vi "Tosca-Compute Histogram.vi"(0 "Results in":T1[](array[typedef]), 5 "family":string, 7 "Result String":string, 9 "Result":T2) -> (4 "Results out":T1[](array[typedef]))   [LabVIEW 2020]
uses:
  Classes/Parameters/Histogram Data.ctl
  Typedefs/Tosca-Trial Result Enum.ctl
  Classes/Parameters/Parameters.lvclass
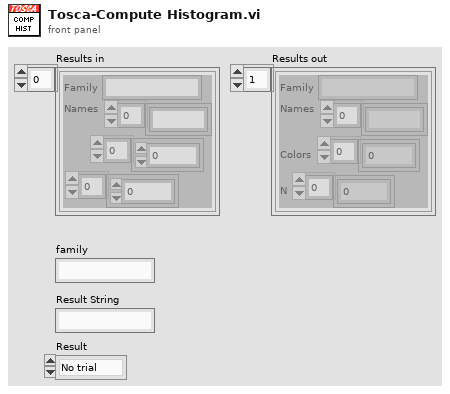
[diagram p1: front panel]
types:
  T1 = typedef "Parameters.lvclass/Histogram Data.ctl" = cluster{"Family":string, "Names":string[], "Colors":u32[], "N":i32[]}
  T2 = typedef "Tosca-Trial Result Enum.ctl" = enum16{"No trial", "Go", "No go", "Error", "Abort"}
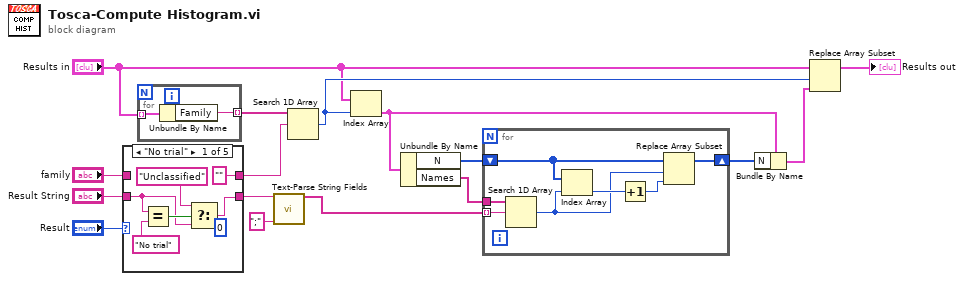
[diagram p0: block diagram]
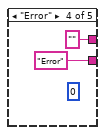
[diagram p4: hidden frame]
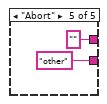
[diagram p5: hidden frame]
diagram:
  n1 = case shown="\"No trial\"" "Result" {
    tunnel: [w20 w23 w25 "Error" ("family") "other" ("family")] -> w6
    tunnel: "family" -> [_ w24 w26 _ _]
    tunnel: ["" ("family") w24 w26 "" ("family") "" ("family")] -> w11
    tunnel: "Result String" -> [w18 w23 w25 _ _]
    frame "No trial" {
      (unwired) i16 0
      n2 = Equal?(x=w18, y="No trial" ("family")) -> (x = y?=w19:bool)
      n3 = Select(t="Unclassified" ("family"), s=w19, f=w18) -> (s? t:f=w20:string)
    }
    frame "Go", Default {
    }
    frame "No go" {
    }
    frame "Error" {
      (unwired) i16 0
    }
    frame "Abort" {
    }
  }
  n4 = for {
    tunnel: "Results in" -> [w32] mode=indexing
    tunnel: [w31] -> w1 mode=indexing
    n5 = Unbundle By Name(w32) -> ("Family"=w31:string)
  }
  n6 = call "Text-Parse String Fields.vi"("String"=w6, "Separator"=";") -> ("Fields"=w4:string[])  [unwired: 8 in, 5 out]
  n7 = Search 1D Array(1D array=w1, element=w11) -> (index of element=w3:i32)  [unwired: 1 in]
  n8 = Index Array(array="Results in", index=w3) -> (element=w9:T1)
  n9 = Unbundle By Name(w9) -> ("N"=w7:i32[], "Names"=w8:string[])
  n10 = for {
    tunnel: w8 -> [w36]
    shift-right: [w39] -> w13
    shift-left: w7 -> [w35]
    tunnel: w4 -> [w33] mode=indexing
    n11 = Search 1D Array(1D array=w36, element=w33) -> (index of element=w34:i32)  [unwired: 1 in]
    n12 = Index Array(array=w35, index=w34) -> (element=w38:i32)
    n13 = Increment(x=w38) -> (x+1=w37:i32)
    n14 = Replace Array Subset(array=w35, new element=w37, index=w34) -> (w39:i32[])
  }
  n15 = Bundle By Name(cluster=w9, "N"=w13) -> (w12:T1)
  n16 = Replace Array Subset(array="Results in", new element=w12, index=w3) -> (→"Results out":T1[])
